vi "Signal from fluke.vi"() -> ()   [LabVIEW 2014]
uses:
  <vilib>/Utility/error.llb/DialogType.ctl
  <instrlib>/Fluke 884X Series/Public/Data/Read (Multiple Points).vi
  <vilib>/Utility/file.llb/Write To Spreadsheet File (DBL).vi
  <instrlib>/Fluke 884X Series/Fluke 884X Series.lvlib
panel:
  out "Signal":dbl
  in  "stop":bool
  in  "Write":bool
  in  "Serial Configuration":T1={"Baud Rate"=9600, "Parity"=0, "Data Bits"=8, "Stop Bits"=10, "Flow Control"=0} {"Flow Control" items=["None", "XON/XOFF", "RTS/CTS", "XON/XOFF & RTS/CTS", "DTR/DSR", "XON/XOFF & DTR/DSR"]; "Stop Bits" items=["1.0"=10, "1.5"=15, "2.0"=20]; "Data Bits" items=["7"=7, "8"=8]; "Parity" items=["None", "Odd", "Even", "Mark", "Space"]; "Baud Rate" items=["300"=300, "600"=600, "1200"=1200, "2400"=2400, "4800"=4800, "9600"=9600, "19200"=19200]}
  in  "VISA resource name":refnum<visa-resource-name>
  in  "Timeout":i32=10000
  in  "Sample Count (10)":i32=10
  in  "Manual Range (1.0)":dbl=1.0
  in  "Auto Range (T:Enable)":bool=TRUE
  in  "Function (0: DC Voltage)":u16(ring) items=["DC Voltage", "AC Voltage", "2 - Wire Resistance", "4 - Wire Resistance", "DC Current", "AC Current", "Frequency", "Period", "Continuity", "Diode Checking", "Temperature", "Capacitance"]
  in  "Manual Resolution (5.5 Digits)":dbl(ring)=5.5 items=["4.5"=4.5, "5.5"=5.5, "6.5"=6.5]
  out "Temperature from Fluke884X":dbl[](graph)
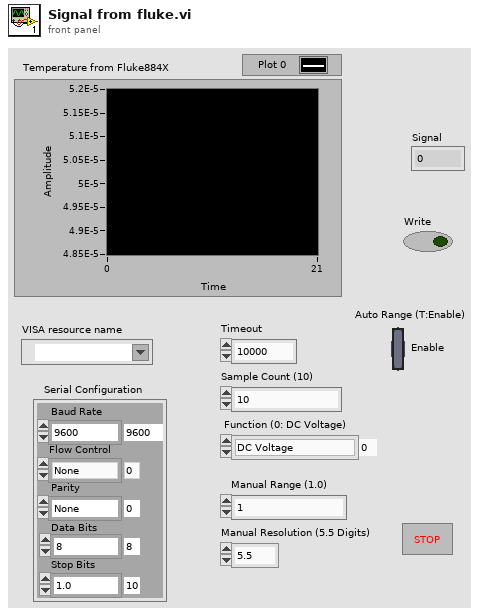
[diagram p1: front panel]
types:
  T1 = cluster{"Baud Rate":u32, "Parity":u16, "Data Bits":u16, "Stop Bits":u16, "Flow Control":u16}
  T2 = typedef "DialogType.ctl" = u16
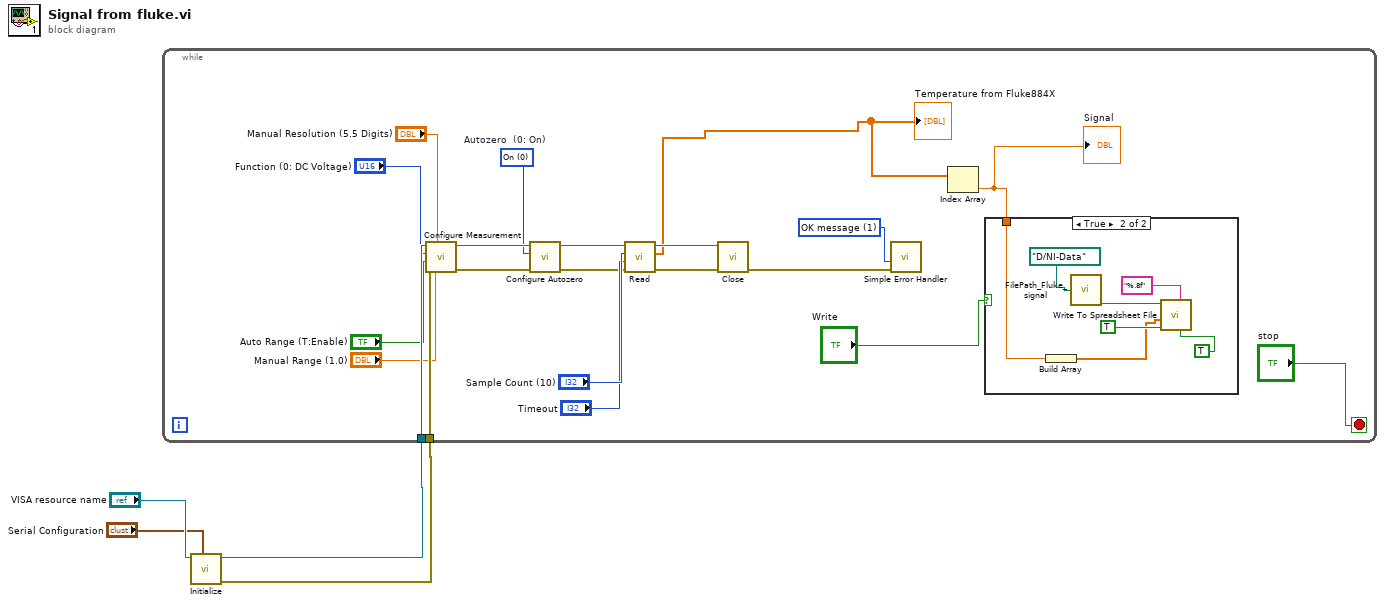
[diagram p0: block diagram]
diagram:
  n1 = call <instrlib>:"Initialize.vi"("Serial Configuration"="Serial Configuration", "VISA resource name"="VISA resource name") -> ("error out"=w1:errorcluster, "VISA resource name out"=w2:refnum<visa-resource-name>)  [unwired: 8 in]
  n2 = while {
    tunnel: w2 -> [w25]
    tunnel: w1 -> [w24]
    stop <- "stop" stop-if-true
    w9 = u16 0 items=["On", "Off", "Once"]  # Autozero  (0: On)
    w23 = T2 1 items=["no dialog", "OK message", "continue or stop message", "OK message + warnings", "continue/stop + warnings"] ("type of dialog (OK msg:1)")
    n3 = call <instrlib>:"Configure Measurement.vi"("Manual Range (1.0)"="Manual Range (1.0)", "Manual Resolution (5.5 Digits)"="Manual Resolution (5.5 Digits)", "error in (no error)"=w24, "Auto Range (T:Enable)"="Auto Range (T:Enable)", "Function (0: DC Voltage)"="Function (0: DC Voltage)", "VISA resource name"=w25) -> ("error out"=w13:errorcluster, "VISA resource name out"=w12:refnum<visa-resource-name>)  [unwired: 4 in]
    n4 = call <instrlib>:"Configure Autozero.vi"("error in (no error)"=w13, "Autozero  (0: On)"=w9, "VISA resource name"=w12) -> ("error out"=w10:errorcluster, "VISA resource name out"=w11:refnum<visa-resource-name>)  [unwired: 7 in]
    n5 = call-poly <instrlib>:"Read.vi"("error in (no error)"=w10, "Timeout (10000 ms)"="Timeout", "Sample Count (1)"="Sample Count (10)", "VISA resource name"=w11) -> ("error out"=w20:errorcluster, "Measurements"=w8:dbl[], "VISA resource name out"=w21:refnum<visa-resource-name>)  [unwired: 5 in]
    "Temperature from Fluke884X" <- w8
    n6 = call <instrlib>:"Close.vi"("error in (no error)"=w20, "VISA resource name"=w21) -> ("error out"=w22:errorcluster)  [unwired: 9 in]
    n7 = call <vilib>:"Simple Error Handler.vi"("type of dialog (OK msg:1)"=w23, "error in (no error)"=w22) -> ()  [unwired: 3 in, 5 out]
    n8 = Index Array(array=w8) -> (element=w5:dbl)  [unwired: 1 in]
    "Signal" <- w5
    n9 = case shown="True" "Write" {
      tunnel: w5 -> [_ w28]
      frame False {
      }
      frame True {
        n10 = Build Array(w28) -> (w27:dbl[])
        n11 = call "FilePath_Fluke_signal.vi"("base folder path"=path "D:/NI-Data") -> ("Signal"=w32:path)  [unwired: 3 out]
        n12 = call-poly <vilib>:"Write To Spreadsheet File.vi"("transpose? (no:F)"=TRUE, "format (%.3f)"="%.8f", "append to file? (new file:F)"=TRUE, "1D data"=w27, "file path (dialog if empty)"=w32) -> ()  [unwired: 1 in, 3 out]
      }
    }
  }
